vi "init.vi"(8 "error in":errorcluster, 10 "TBM module configuration in":refnum<class "TBM module configuration.lvclass">, 11 "J1939 runtime in":refnum<class "J1939 runtime.lvclass">) -> (0 "error out":errorcluster, 1 "data allocations":T1, 2 "execution settings":T4, 3 "J1939 runtime out":refnum<class "J1939 runtime.lvclass">)   [LabVIEW 2013, in "J1939 runtime.lvclass"]
doc: "Provides an interface for initializing a module at runtime. While this interface performs no operations, a child should provide an override which may open any necessary references or sessions, allocate necessary memory, and perform any final configuration validataion before providing the full configuration <b>execution data</b> to the calling process."
uses:
  J1939 runtime.lvclass
  <vilib>/NI/Tag Bus Module Framework/module configuration/TBM module configuration.lvclass
  <vilib>/NI/Tag Bus Module Framework/runtime/execution settings.ctl
  <vilib>/NI/Tag Bus Module Framework/channel/data tables.ctl
  <vilib>/NI/Tag Bus/dictionary/data dictionary.lvclass
  <vilib>/NI/Tag Bus/dictionary table pair.ctl
  <vilib>/NI/Tag Bus/table/data table.ctl
  configuration/J1939 configuration.lvclass
  configuration/J1939 configuration.lvclass/J1939 configuration.ctl
  J1939 runtime.lvclass/J1939 runtime.ctl
  configuration/Read Lines.vi
  <vilib>/NI/Tag Bus Module Framework/channel/TBM channel.lvclass
  <vilib>/NI/Tag Bus Module Framework/runtime/TBM module execution interface.lvclass
  <vilib>/NI/Tag Bus/tag bus.lvlib
  <vilib>/NI/Tag Bus/table/data table.lvlib
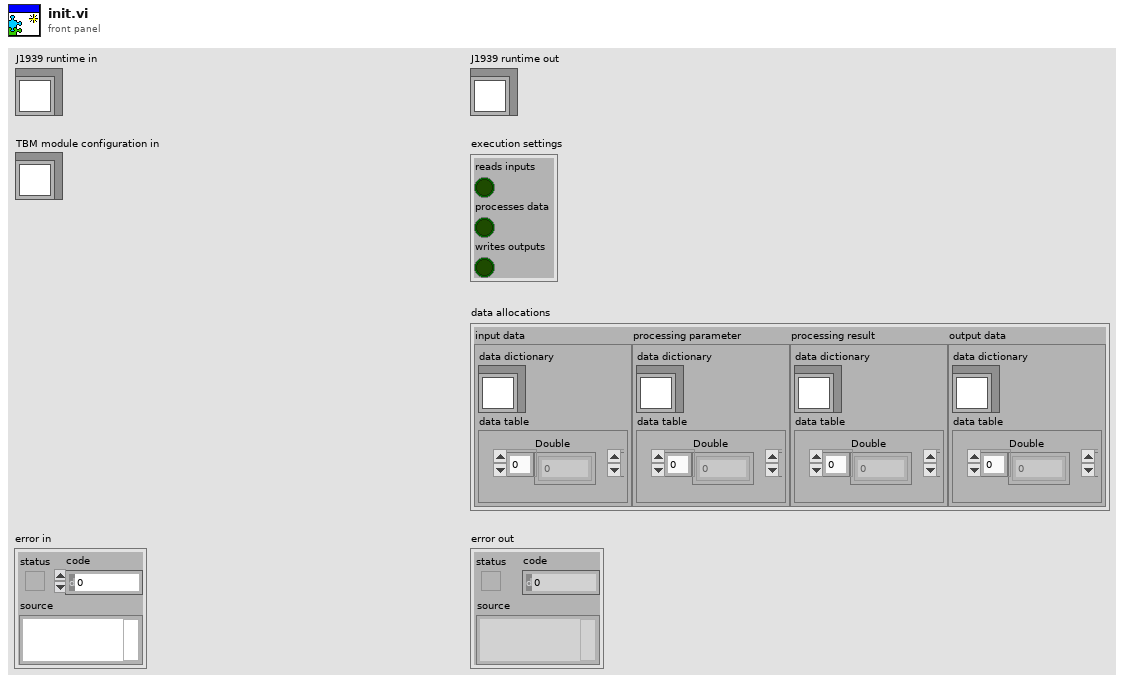
[diagram p1: front panel]
types:
  T1 = typedef "TBM channel.lvclass/data tables.ctl" = cluster{"input data":T2, "processing parameter":T2, "processing result":T2, "output data":T2}
  T2 = typedef "tag bus.lvlib/dictionary table pair.ctl" = cluster{"data dictionary":refnum<class "data dictionary.lvclass">, "data table":T3}
  T3 = typedef "tag bus.lvlib/data table.lvlib/data table.ctl" = cluster{"Double":dbl[], "Single":sgl[], "I64":i64[], "I32":i32[], "I16":i16[], "I8":i8[], "U64":u64[], "U32":u32[], "U16":u16[], "U8":u8[], "Boolean":bool[], "String":string[], "Array of Double":cluster{"DBL Array":dbl[]}[], "Array of Single":cluster{"SGL Array":sgl[]}[], "Array of I64":cluster{"I64 Array":i64[]}[], "Array of I32":cluster{"I32 Array":i32[]}[], "Array of I16":cluster{"I16 Array":i16[]}[], "Array of I8":cluster{"I8 Array":i8[]}[], "Array of U64":cluster{"U64 Array":u64[]}[], "Array of U32":cluster{"U32 Array":u32[]}[], "Array of U16":cluster{"U16 Array":u16[]}[], "Array of U8":cluster{"U8 Array":u8[]}[], "Array of Boolean":cluster{"Boolean Array":bool[]}[], "Array of String":cluster{"String Array":string[]}[]}
  T4 = typedef "TBM module execution interface.lvclass/execution settings.ctl" = cluster{"reads inputs":bool, "processes data":bool, "writes outputs":bool}
  T5 = typedef "J1939 configuration.lvclass/Line.ctl" = cluster{"channel":refnum<class "TBM channel.lvclass">, "XNET Signal":refnum<k21>}
  T6 = typedef "J1939.lvlib/Signal Mapping.ctl" = cluster{"data type":T7, "index":i32}
  T7 = typedef "tag bus.lvlib/tag descriptor.lvclass/Data Type.ctl" = enum16{"Double", "Single", "I64", "I32", "I16", "I8", "U64", "U32", "U16", "U8", "Boolean", "String", "Array of Double", "Array of Single", "Array of I64", "Array of I32", "Array of I16", "Array of I8", "Array of U64", "Array of U32", "Array of U16", "Array of U8", "Array of Boolean", "Array of String"}
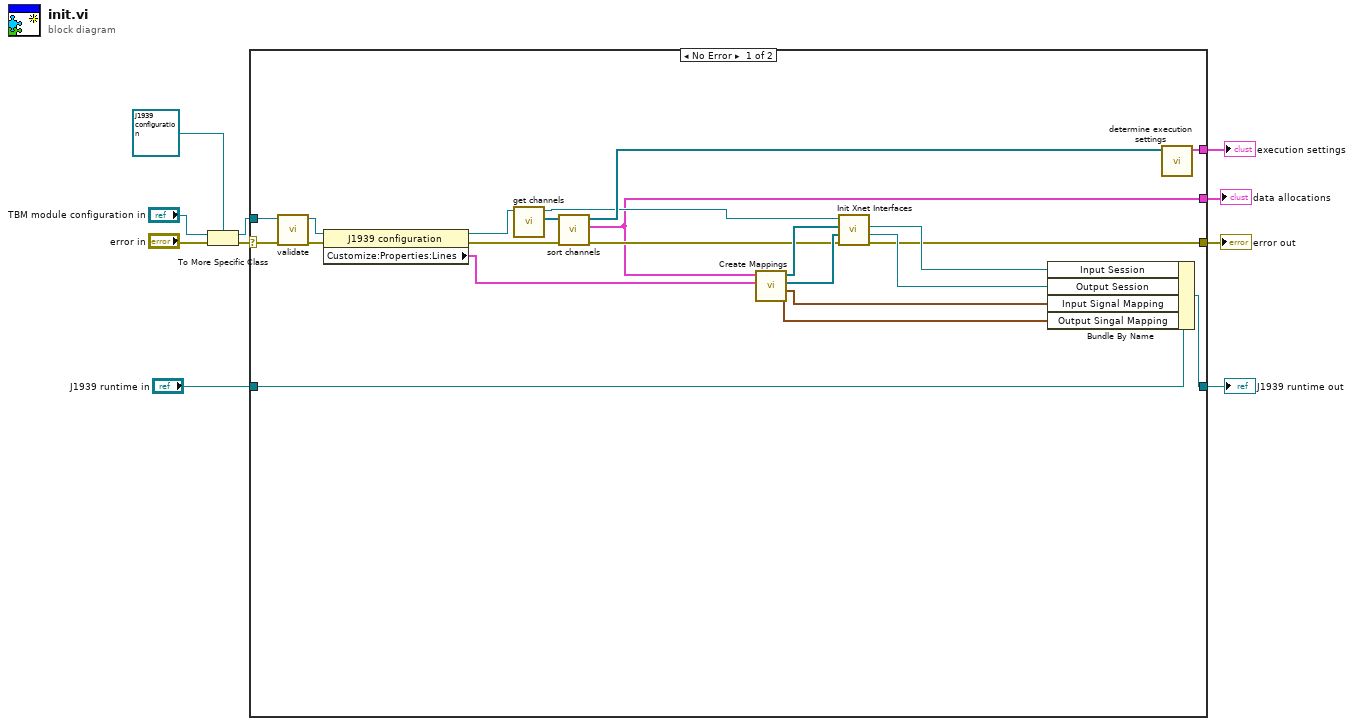
[diagram p0: block diagram]
diagram:
  n1 = To More Specific Class(target class=refnum<class "J1939 configuration.lvclass"> refnum ("Synchronous module configuration"), reference="TBM module configuration in", error in="error in") -> (specific class reference=w9:refnum<class "J1939 configuration.lvclass">, error out=w10:errorcluster)
  n2 = case shown="No Error" w10 {
    selector: w10 -> [w30 w33]
    tunnel: w9 -> [w29 _]
    tunnel: "J1939 runtime in" -> [w25 w34]
    tunnel: [w24 w34] -> w4
    tunnel: [w17 w33] -> w3
    tunnel: [w13 _] -> w1
    tunnel: [w32 _] -> w2
    frame No Error {
      n3 = call-dynamic "validate.vi"("error in"=w30, "J1939 configuration in"=w29) -> ("error out"=w26:errorcluster, "J1939 configuration out"=w28:refnum<class "J1939 configuration.lvclass">)  [unwired: 8 in]
      n4 = property class="J1939 configuration"(reference=w28, error in=w26) -> (reference out=w23:refnum<class "J1939 configuration.lvclass">, error out=w16:errorcluster, "Customize:Properties:Lines"=w27:T5[])
      n5 = call-dynamic "get channels.vi"("J1939 configuration in"=w23) -> ("channels"=w14:refnum<class "TBM channel.lvclass">[], "J1939 configuration out"=w15:refnum<class "J1939 configuration.lvclass">)  [unwired: 9 in]
      n6 = call <vilib>:"sort channels.vi"("error in"=w16, "channels in"=w14) -> ("error out"=w18:errorcluster, "data allocations"=w13:T1, "channels out"=w31:refnum<class "TBM channel.lvclass">[])  [unwired: 7 in]
      n7 = call "Create Mappings.vi"("Lines"=w27, "data allocations"=w13) -> ("Output Mapping"=w11:T6[], "Input Mapping"=w12:T6[], "Output Singals"=w21:refnum<k21>[], "Input Singals"=w22:refnum<k21>[])  [unwired: 6 in]
      n8 = call "Init Xnet Interfaces.vi"("error in (no error)"=w18, "Output Singals"=w21, "Input Signals"=w22, "Config In"=w15) -> ("error out"=w17:errorcluster, "Output Session"=w19:refnum<k21>, "Input Session"=w20:refnum<k21>)  [unwired: 4 in, 1 out]
      n9 = Bundle By Name(cluster=w25, "Input Session"=w20, "Output Session"=w19, "Input Signal Mapping"=w12, "Output Singal Mapping"=w11) -> (w24:refnum<class "J1939 runtime.lvclass">)
      n10 = call <vilib>:"determine execution settings.vi"("channels"=w31) -> ("execution settings"=w32:T4)  [unwired: 10 in]
    }
    frame Error {
    }
  }
  "error out" <- w3
  "J1939 runtime out" <- w4
  "execution settings" <- w2
  "data allocations" <- w1
